vi "DataLog Append Points To Log.vi"(0 "tag log directory":path, 7 "points":T1[](array[typedef]) {"value" format="%.3e"; "time" format="%<%H:%M:%S%2u\n%Y/%m/%d>T"}, 11 "error in (no error)":errorcluster) -> (4 "dup tag log directory":path, 15 "error out":errorcluster)   [LabVIEW 2012]
doc: "Append points to the log. The write is broken up if a chunk boundary is crossed. When a log file reaches its chunk content limit, an additional log file is created. When the last chunk is partially written to, it is padded up to the chunk length unless it is the very first chunk of the log. This causes logs holding more than one chunk of data to grow in chunk-sized steps. This results in some storage overhead but helps filesystem avoid fragmentation and makes it unlikely that a chunk is distributed across the physical disk, which should speed up reads.\n\nBy waiting until the last chunk has been successfully written before updating the write index, the composite file I/O is turned into a transaction since the write index is used during reads as a bound to the available data. It is therefore allowable to retry this VI when it fails."
uses:
  typedefs/clusters/t_DataLog Point.ctl
  glb_DataLog MCVD.vi
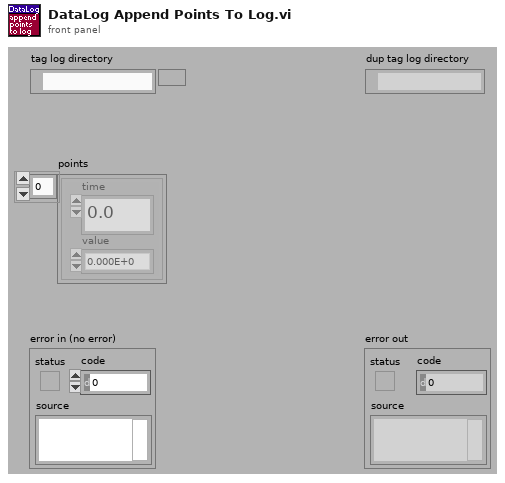
[diagram p1: front panel]
types:
  T1 = typedef "t_DataLog Point.ctl" = cluster{"time":dbl, "value":dbl}
  T2 = enum16{"deny read/write", "deny write-only", "deny none"}
  T3 = enum16{"read/write", "read-only", "write-only", "write-only (truncate)"}
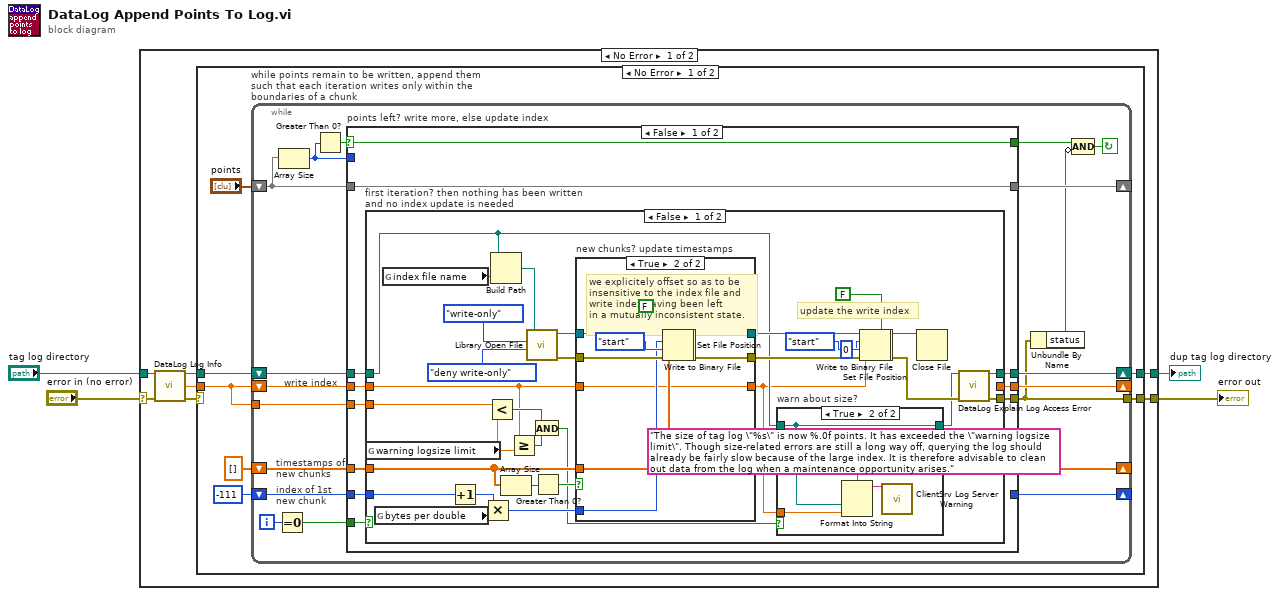
[diagram p0: block diagram]
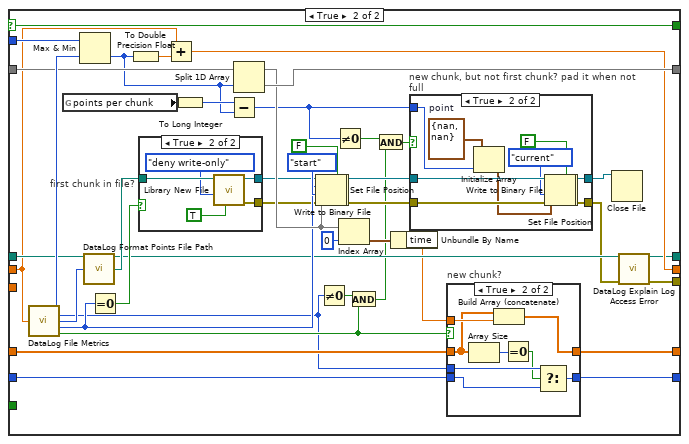
[diagram p5: hidden frame]
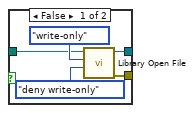
[diagram p8: hidden frame]
diagram:
  n1 = case shown="No Error" "error in (no error)" {
    selector: "error in (no error)" -> [w11 w183]
    tunnel: [w8 w183] -> w4
    tunnel: "tag log directory" -> [w10 w182]
    tunnel: [w7 w182] -> w1
    frame No Error {
      n2 = call "DataLog Log Info.vi"("tag log directory"=w10, "error in (no error)"=w11) -> ("dup tag log directory"=w6:path, "size"=w9:dbl, "error out"=w5:errorcluster)  [unwired: 10 in, 1 out]
      n3 = case shown="No Error" w5 {
        selector: w5 -> [_ w181]
        tunnel: w9 -> [w12 _]
        tunnel: [w13 w181] -> w8
        tunnel: [w14 w180] -> w7
        tunnel: w6 -> [w17 w180]
        frame No Error {
          n4 = while "while points remain to be written, append them such that each iteration writes only within the boundaries of a chunk" {
            shift-right: [w36] -> _
            shift-left: "points" -> [w35]
            shift-right: [w27] -> _
            shift-left: w12 -> [w37]
            shift-right: [w28] -> w14
            shift-left: w17 -> [w30]
            tunnel: [w26] -> w13
            shift-right: [w23] -> _
            shift-left: -111 ("chunk index") -> [w22]
            shift-right: [w21] -> _
            shift-left: dbl[] [] -> [w20]
            tunnel: w12 -> [w19]
            i -> [w25]
            stop <- w33 continue-if-true
            # "timestamps of\nnew chunks"
            # "index of 1st\nnew chunk"
            # "write index"
            n5 = Equal To 0?(x=w25) -> (x = 0?=w24:bool)
            n6 = Array Size(array=w35) -> (size(s)=w29:i32)
            n7 = Greater Than 0?(x=w29) -> (x > 0?=w34:bool)
            n8 = case "points left? write more, else update index" shown="False" w34 {
              selector: w34 -> [w47 w142]
              tunnel: w37 -> [w42 w133]
              tunnel: w35 -> [w48 w144]
              tunnel: [w48 w143] -> w36
              tunnel: [w41 w109] -> w26
              tunnel: [w47 w142] -> w31
              tunnel: w30 -> [w45 w135]
              tunnel: w29 -> [_ w146]
              tunnel: [w44 w110] -> w28
              tunnel: [w43 w137] -> w27
              tunnel: w24 -> [w46 _]
              tunnel: [_ w106] -> w23
              tunnel: w22 -> [w40 w107]
              tunnel: [_ w112] -> w21
              tunnel: w20 -> [w39 w111]
              tunnel: w19 -> [w38 _]
              frame False {
                n9 = case "first iteration? then nothing has been written and no index update is needed" shown="False" w46 {
                  tunnel: [w74 w102] -> w44
                  tunnel: w45 -> [w54 w102]
                  tunnel: w42 -> [w57 w101]
                  tunnel: [_ w101] -> w43
                  tunnel: [w75 _] -> w41
                  tunnel: w40 -> [w65 _]
                  tunnel: w39 -> [w62 _]
                  tunnel: w38 -> [w58 _]
                  frame False {
                    # "update the write index"
                    n10 = global read "glb_DataLog MCVD.vi" "warning logsize limit"() -> (w59:dbl)
                    n11 = global read "glb_DataLog MCVD.vi" "bytes per double"() -> (w72:i32)
                    n12 = global read "glb_DataLog MCVD.vi" "index file name"() -> (w81:string)
                    n13 = Increment(x=w65) -> (x+1=w73:i32)
                    n14 = Multiply(x=w73, y=w72) -> (x*y=w64:i32)
                    n15 = Less?(x=w58, y=w59) -> (x < y?=w61:bool)
                    n16 = Build Path(base path=w54, name or relative path=w81) -> (appended path=w78:path)
                    n17 = Array Size(array=w62) -> (size(s)=w63:i32)
                    n18 = Greater Or Equal?(x=w57, y=w59) -> (x >= y?=w60:bool)
                    n19 = call "Library Open File.vi"("deny mode (deny none)"=T2."deny write-only" ("deny mode (2)"), "open mode (read/write)"=T3."write-only" ("open mode (0)"), "file path"=w78) -> ("error out"=w77:errorcluster, "refnum"=w76:refnum<file>)  [unwired: 3 in]
                    n20 = And(x=w61, y=w60) -> (x .and. y?=w55:bool)
                    n21 = Greater Than 0?(x=w63) -> (x > 0?=w56:bool)
                    n22 = case "new chunks? update timestamps" shown="True" w56 {
                      tunnel: w77 -> [w88 w100]
                      tunnel: w76 -> [w89 w99]
                      tunnel: [w89 w97] -> w71
                      tunnel: [w88 w96] -> w70
                      tunnel: w62 -> [_ w95]
                      tunnel: w64 -> [_ w94]
                      tunnel: [w87 w93] -> w52
                      tunnel: w57 -> [w87 w93]
                      frame False {
                      }
                      frame True {
                        # "we explicitely offset so as to be\ninsensitive to the index file and\nwrite index having been left\nin a mutually inconsistent state."
                        n23 = Set File Position(offset (in bytes) (0)=w94, refnum=w99, from (0:start)=enum16{"start", "end", "current"}."start" ("pos mode (0:2)"), error in=w100) -> (refnum out=w92:refnum<file>, error out=w91:errorcluster)
                        n24 = Write to Binary File(file (use dialog)=w92, data=w95, error in=w91, 5:FALSE ("prepend array or string size? (T)")) -> (refnum out=w97:refnum<file>, error out=w96:errorcluster)  [unwired: 2 in, 1 out]
                      }
                    }
                    n25 = case "warn about size?" shown="True" w55 {
                      tunnel: w54 -> [w82 w86]
                      tunnel: [w82 w86] -> w53
                      tunnel: w52 -> [_ w83]
                      frame False {
                      }
                      frame True {
                        n26 = Format Into String(format string="The size of tag log \"%s\" is now %.0f points. It has exceeded the \"warning logsize limit\". Though size-related errors are still a long way off, querying the log should already be fairly slow because of the large index. It is therefore advisable to clean out data from the log when a maintenance opportunity arises.", w86, w83) -> (resulting string=w85:string)  [unwired: 2 in, 1 out]
                        n27 = call "ClientSrv Log Server Warning.vi"("message (use cluster)"=w85) -> ()  [unwired: 15 in]
                      }
                    }
                    n28 = Set File Position(offset (in bytes) (0)=0 ("pos offset (0)"), refnum=w71, from (0:start)=enum16{"start", "end", "current"}."start" ("pos mode (0:2)"), error in=w70) -> (refnum out=w51:refnum<file>, error out=w50:errorcluster)
                    n29 = Write to Binary File(file (use dialog)=w51, data=w52, error in=w50, 5:FALSE ("prepend array or string size? (T)")) -> (refnum out=w68:refnum<file>, error out=w69:errorcluster)  [unwired: 2 in, 1 out]
                    n30 = Close File(refnum=w68) -> ()  [unwired: 1 in, 2 out]
                    n31 = call "DataLog Explain Log Access Error.vi"("tag log directory"=w53, "error in"=w69) -> ("dup tag log directory"=w74:path, "error out"=w75:errorcluster)  [unwired: 12 in]
                  }
                  frame True {
                  }
                }
              }
              frame True {
                n32 = call "DataLog File Metrics.vi"("point index"=w133) -> ("points left in chunk"=w145:i32, "chunk index"=w108:i32, "log file index"=w136:i32, "log file offset"=w132:i32, "at chunk boundary?"=w114:bool)  [unwired: 9 in, 1 out]
                n33 = global read "glb_DataLog MCVD.vi" "points per chunk"() -> (w126:dbl)
                n34 = Max & Min(x=w146, y=w145) -> (min(x,y)=w124:i32)  [unwired: 1 out]
                n35 = call "DataLog Format Points File Path.vi"("tag log directory"=w135, "log file index"=w136) -> ("dup tag log directory"=w127:path, "log file path"=w130:path)  [unwired: 12 in]
                n36 = Equal To 0?(x=w132) -> (x = 0?=w131:bool)
                n37 = To Double Precision Float(number=w124) -> (double precision float=w134:dbl)
                n38 = case "first chunk in file?" shown="True" w131 {
                  tunnel: w130 -> [w172 w179]
                  tunnel: [w171 w177] -> w129
                  tunnel: [w170 w178] -> w128
                  frame False {
                    n39 = call "Library Open File.vi"("deny mode (deny none)"=T2."deny write-only" ("deny mode (2)"), "open mode (read/write)"=T3."write-only" ("open mode (0)"), "file path"=w172) -> ("error out"=w171:errorcluster, "refnum"=w170:refnum<file>)  [unwired: 3 in]
                  }
                  frame True {
                    n40 = call "Library New File.vi"("overwrite (F)"=TRUE, "deny mode (deny none)"=T2."deny write-only" ("deny mode (2)"), "file path"=w179) -> ("error out"=w177:errorcluster, "refnum"=w178:refnum<file>)  [unwired: 7 in]
                  }
                }
                n41 = Add(x=w133, y=w134) -> (x+y=w137:dbl)
                n42 = To Long Integer(number=w126) -> (32bit integer=w125:i32)
                n43 = Subtract(x=w125, y=w124) -> (x-y=w116:i32)
                n44 = Split 1D Array(array=w144, index=w124) -> (first subarray=w140:T1[], second subarray=w143:T1[])
                n45 = Set File Position(offset (in bytes) (0)=w132, refnum=w128, from (0:start)=enum16{"start", "end", "current"}."start" ("pos mode (0:2)"), error in=w129) -> (refnum out=w105:refnum<file>, error out=w104:errorcluster)
                n46 = Write to Binary File(file (use dialog)=w105, data=w140, error in=w104, 5:FALSE ("prepend array or string size? (T)")) -> (refnum out=w121:refnum<file>, error out=w122:errorcluster)  [unwired: 2 in, 1 out]
                n47 = Not Equal To 0?(x=w108) -> (x != 0?=w123:bool)
                n48 = Not Equal To 0?(x=w116) -> (x != 0?=w115:bool)
                n49 = Index Array(array=w140, index=0) -> (element=w138:T1)
                n50 = And(x=w123, y=w114) -> (x .and. y?=w117:bool)
                n51 = And(x=w115, y=w117) -> (x .and. y?=w118:bool)
                n52 = Unbundle By Name(w138) -> ("time"=w113:dbl)
                n53 = case "new chunk, but not first chunk? pad it when not full" shown="True" w118 {
                  tunnel: w122 -> [w157 w168]
                  tunnel: w121 -> [w158 w167]
                  tunnel: w116 -> [_ w166]
                  tunnel: [w158 w163] -> w120
                  tunnel: [w157 w162] -> w119
                  frame False {
                  }
                  frame True {
                    w169 = T1 {"time"=nan, "value"=nan}  # point
                    n54 = Initialize Array(w169, w166) -> (w165:T1[])
                    n55 = Set File Position(refnum=w167, from (0:start)=enum16{"start", "end", "current"}."current" ("pos mode (0:2)"), error in=w168) -> (refnum out=w161:refnum<file>, error out=w160:errorcluster)  [unwired: 1 in]
                    n56 = Write to Binary File(file (use dialog)=w161, data=w165, error in=w160, 5:FALSE ("prepend array or string size? (T)")) -> (refnum out=w163:refnum<file>, error out=w162:errorcluster)  [unwired: 2 in, 1 out]
                  }
                }
                n57 = case "new chunk?" shown="True" w114 {
                  tunnel: w113 -> [_ w156]
                  tunnel: [w148 w155] -> w112
                  tunnel: w111 -> [w148 w151]
                  tunnel: w108 -> [_ w154]
                  tunnel: w107 -> [w147 w152]
                  tunnel: [w147 w153] -> w106
                  frame False {
                  }
                  frame True {
                    n58 = Array Size(array=w151) -> (size(s)=w150:i32)
                    n59 = Build Array (concatenate)(w151, w156) -> (w155:dbl[])
                    n60 = Equal To 0?(x=w150) -> (x = 0?=w149:bool)
                    n61 = Select(t=w154, s=w149, f=w152) -> (s? t:f=w153:i32)
                  }
                }
                n62 = Close File(refnum=w120) -> ()  [unwired: 1 in, 2 out]
                n63 = call "DataLog Explain Log Access Error.vi"("tag log directory"=w127, "error in"=w119) -> ("dup tag log directory"=w110:path, "error out"=w109:errorcluster)  [unwired: 12 in]
              }
            }
            n64 = Unbundle By Name(w26) -> ("status"=w32:bool)
            n65 = Compound Arithmetic op=AND(w31, invert w32) -> (w33:bool)
          }
        }
        frame Error {
        }
      }
    }
    frame Error {
    }
  }
  "error out" <- w4
  "dup tag log directory" <- w1
